vi "event_occurrances2.vi"() -> ()   [LabVIEW 2019]
panel:
  out "Numeric 2":i32
  out "iter2":i32
  out "Numeric":i32
  out "iter":i32
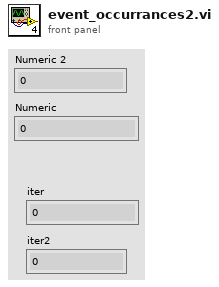
[diagram p1: front panel]
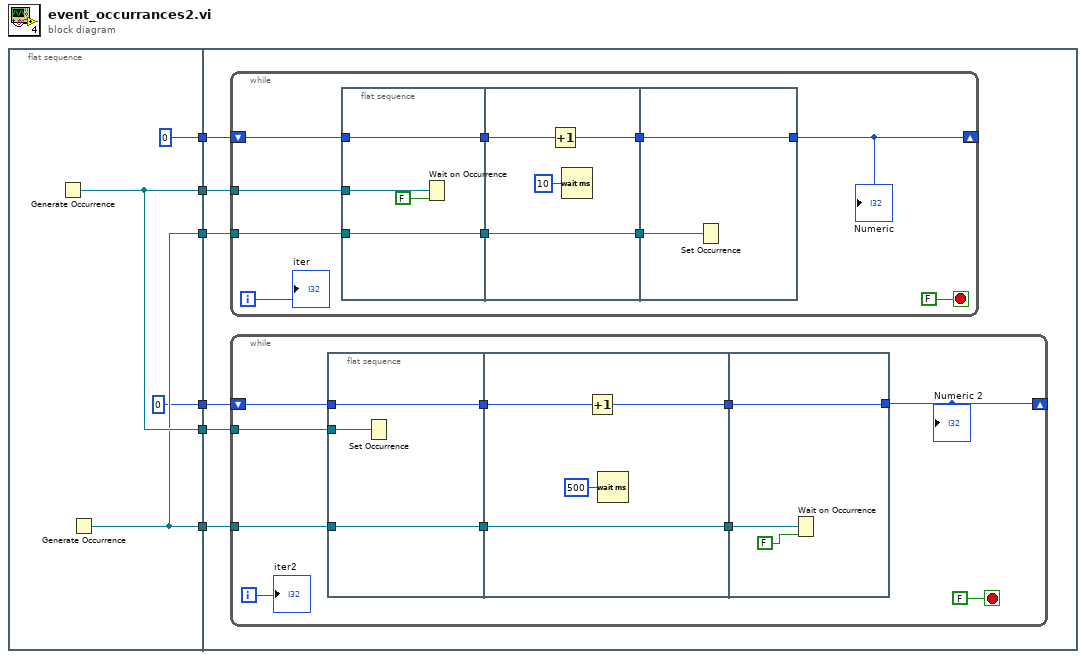
[diagram p0: block diagram]
diagram:
  n1 = flat-sequence {
    tunnel: [w10] -> w6
    tunnel: [w10] -> w5
    tunnel: [0] -> w4
    tunnel: [w8] -> w3
    tunnel: [w8] -> w2
    tunnel: [0] -> w1
    tunnel: w6 -> [w16]
    tunnel: w5 -> [w15]
    tunnel: w4 -> [w14]
    tunnel: w3 -> [w13]
    tunnel: w2 -> [w12]
    tunnel: w1 -> [w11]
    frame #0 {
      n2 = Generate Occurrence() -> (w10:refnum<k4>)
      n3 = Generate Occurrence() -> (w8:refnum<k4>)
    }
    frame #1 {
      n4 = while {
        tunnel: w16 -> [w46]
        shift-right: [w41] -> _
        shift-left: w14 -> [w42]
        tunnel: w12 -> [w39]
        i -> [w44]
        stop <- FALSE stop-if-true
        n5 = flat-sequence {
          tunnel: w46 -> [w50]
          tunnel: [w49] -> w43
          tunnel: w42 -> [w49]
          tunnel: w39 -> [w48]
          tunnel: [w48] -> w38
          tunnel: w43 -> [w54]
          tunnel: [w53] -> w40
          tunnel: w38 -> [w52]
          tunnel: [w52] -> w37
          tunnel: [w56] -> w41
          tunnel: w40 -> [w56]
          tunnel: w37 -> [w55]
          frame #0 {
            n6 = Wait on Occurrence(1:FALSE ("ignore previous (T)"), 2:w50) -> ()  [unwired: 1 in, 1 out]
          }
          frame #1 {
            n7 = Increment(x=w54) -> (x+1=w53:i32)
            n8 = Wait (ms)(milliseconds to wait=u32 10) -> ()  [unwired: 1 out]
          }
          frame #2 {
            n9 = Set Occurrence(w55) -> ()
          }
        }
        "iter" <- w44
        "Numeric" <- w41
      }
      n10 = while {
        tunnel: w15 -> [w25]
        tunnel: w13 -> [w23]
        shift-right: [w17] -> _
        shift-left: w11 -> [w21]
        i -> [w24]
        stop <- FALSE stop-if-true
        n11 = flat-sequence {
          tunnel: w25 -> [w28]
          tunnel: w23 -> [w29]
          tunnel: [w29] -> w22
          tunnel: w21 -> [w27]
          tunnel: [w27] -> w19
          tunnel: w22 -> [w33]
          tunnel: [w33] -> w20
          tunnel: w19 -> [w31]
          tunnel: [w30] -> w18
          tunnel: w20 -> [w36]
          tunnel: w18 -> [w35]
          tunnel: [w35] -> w17
          frame #0 {
            n12 = Set Occurrence(w28) -> ()
          }
          frame #1 {
            n13 = Increment(x=w31) -> (x+1=w30:i32)
            n14 = Wait (ms)(milliseconds to wait=u32 500) -> ()  [unwired: 1 out]
          }
          frame #2 {
            n15 = Wait on Occurrence(1:FALSE ("ignore previous (T)"), 2:w36) -> ()  [unwired: 1 in, 1 out]
          }
        }
        "iter2" <- w24
        "Numeric 2" <- w17
      }
    }
  }
